vi "GateDelay_Engine_V1.vi"(0 "Port Array":refnum<visa-resource-name>[](array[refnum]), 2 "DelayGate Action":T1=enum."Exit", 5 "Device Index":i32, 9 "Delay Value (steps)":string) -> (8 "Current Delays":i32[][](array[numeric]))   [LabVIEW 2014]
uses:
  GateDelayAction_TypeDef.ctl
  <vilib>/Instr/_visa.llb/VISA Open Access Mode.ctl
  <vilib>/Instr/_visa.llb/VISA Configure Serial Port (Instr).vi
  <vilib>/Instr/_visa.llb/VISA Find Search Mode.ctl
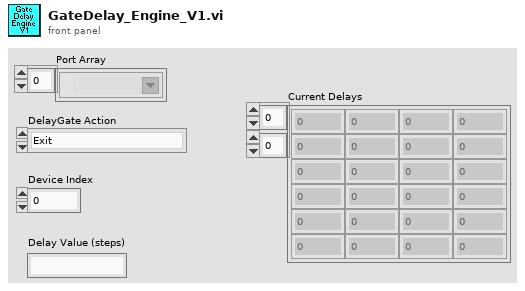
[diagram p1: front panel]
types:
  T1 = typedef "GateDelayAction_TypeDef.ctl" = enum16{"Set Laser Delay", "Set Window Delay", "Set Window Width", "Get Delays", "Exit", "CloseConnections", "Initialize"}
  T2 = typedef "VISA Find Search Mode.ctl" = u32
  T3 = typedef "VISA Open Access Mode.ctl" = u32
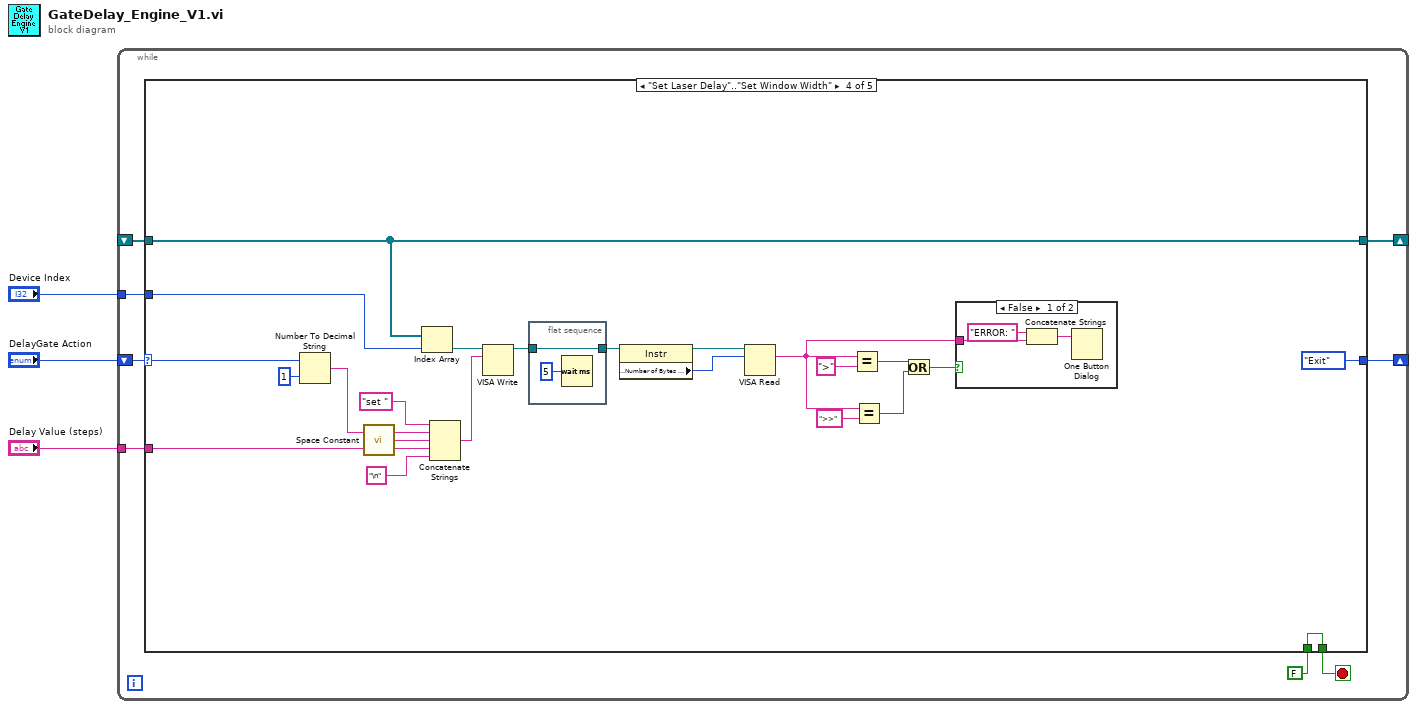
[diagram p0: block diagram]
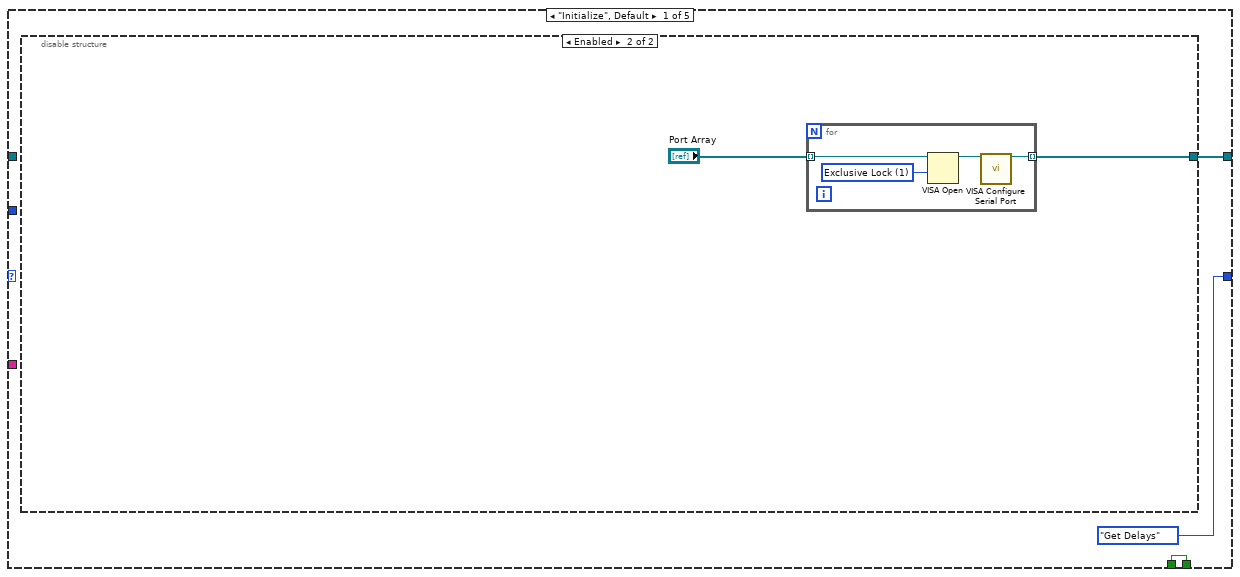
[diagram p2: hidden frame]
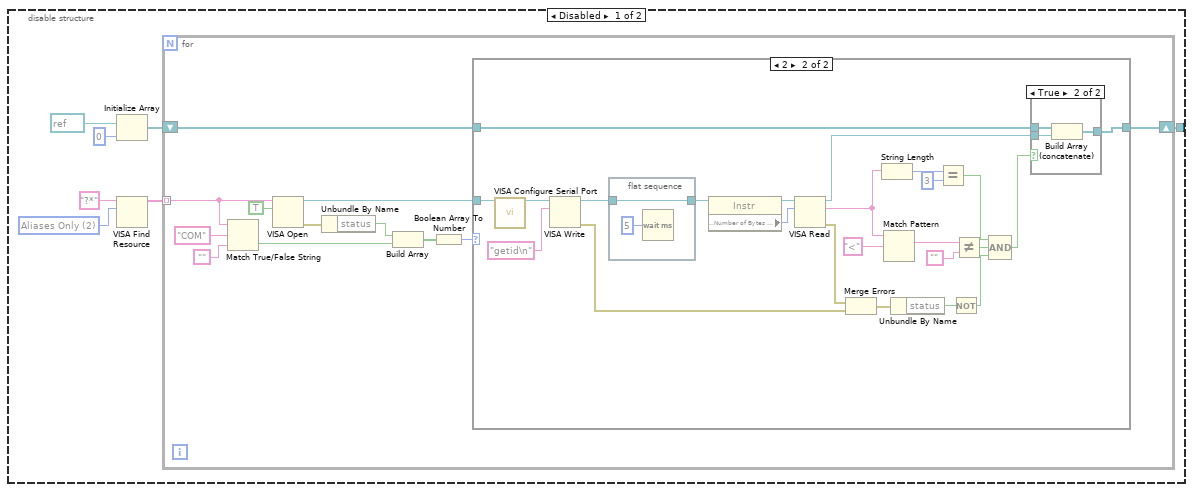
[diagram p3: hidden frame]
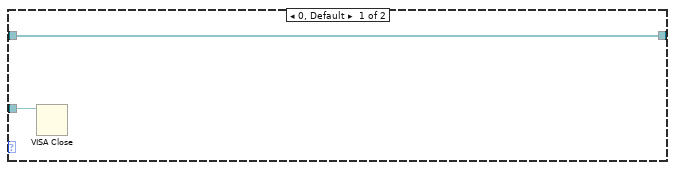
[diagram p4: hidden frame]
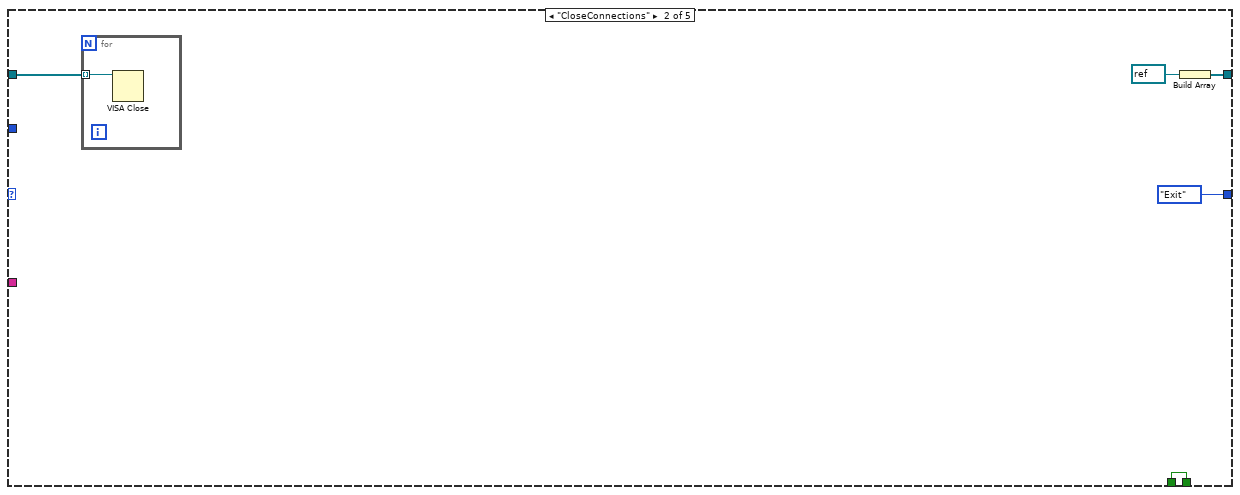
[diagram p6: hidden frame]
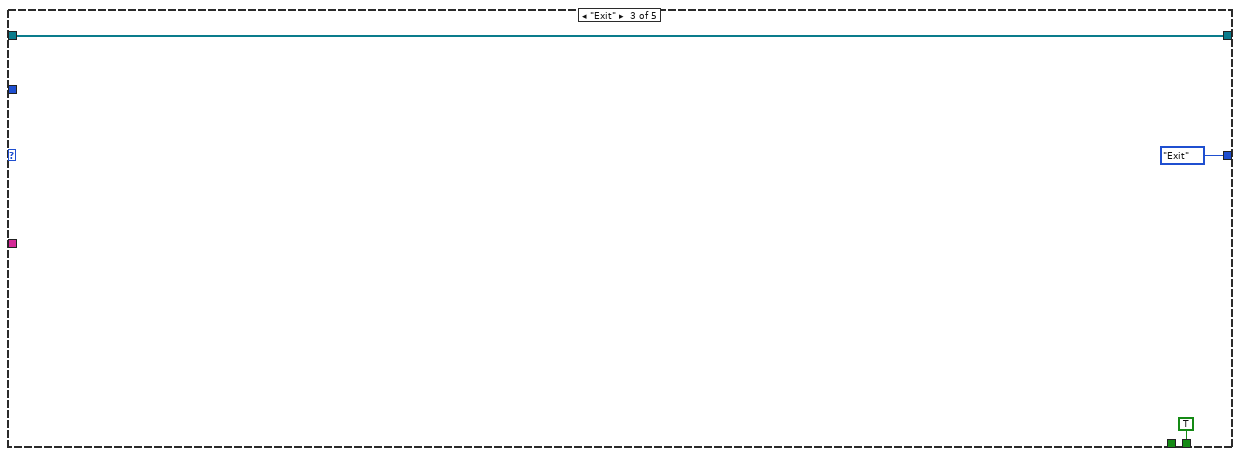
[diagram p7: hidden frame]
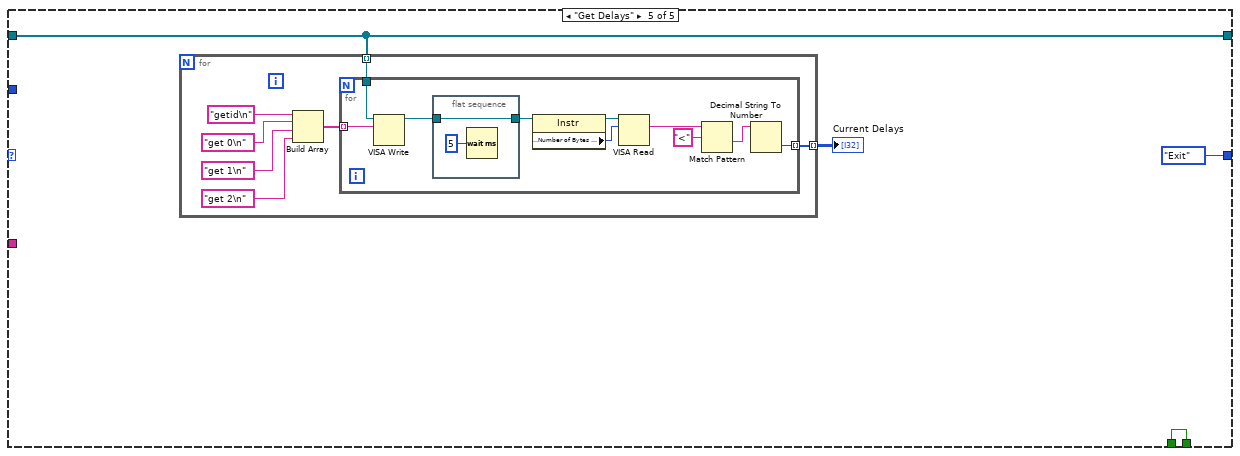
[diagram p9: hidden frame]
diagram:
  n1 = while {
    shift-right: [w8] -> _
    shift-left: "DelayGate Action" -> [w9]
    shift-right: [w11] -> _
    shift-left: _ -> [w10]
    tunnel: "Device Index" -> [w5]
    tunnel: "Delay Value (steps)" -> [w4]
    stop <- w6 stop-if-true
    n2 = case shown="\"Set Laser Delay\"..\"Set Window Width\"" w9 {
      selector: w9 -> [_ _ _ w89 _]
      tunnel: [w14 w73 w78 w103 w110] -> w11
      tunnel: w10 -> [_ w76 w78 w103 w110]
      tunnel: [GateDelayAction_TypeDef."Get Delays" ("Enum") GateDelayAction_TypeDef."Exit" ("Enum") GateDelayAction_TypeDef."Exit" ("Enum") GateDelayAction_TypeDef."Exit" ("Enum") GateDelayAction_TypeDef."Exit" ("Enum")] -> w8
      tunnel: FALSE -> [w12 w72 _ w93 w112]
      tunnel: [w12 w72 TRUE w93 w112] -> w6
      tunnel: w5 -> [_ _ _ w86 _]
      tunnel: w4 -> [_ _ _ w101 _]
      frame "Initialize", Default {
        n3 = disable-structure shown="Enabled" {
          disable-tunnel: [w15 w67] -> w14
          frame Disabled {
            w20 = T2 2 items=["Canonical Names Only"=0, "Aliases Only"=2, "Include Matching Aliases"=3, "Include All Aliases"=4] ("Search Mode")
            n4 = Initialize Array(refnum<visa-resource-name> refnum ("VISA resource name out"), 0 ("dimension size")) -> (w16:refnum<visa-resource-name>[])
            n5 = VISA Find Resource(10:w20, 11:"?*" ("expression (\"?*\")")) -> (3:w19:string[])  [unwired: 1 in, 2 out]
            n6 = for {
              tunnel: w19 -> [w30] mode=indexing
              shift-right: [w23] -> w15
              shift-left: w16 -> [w24]
              n7 = Match True/False String(2:"", 3:"COM" ("true string"), 4:w30) -> (0:w28:bool)  [unwired: 1 out]
              n8 = VISA Open(duplicate session (F)=TRUE, VISA resource name=w30) -> (VISA resource name=w25:refnum<visa-resource-name>, error out=w31:errorcluster)  [unwired: 3 in]
              n9 = Unbundle By Name(w31) -> ("status"=w29:bool)
              n10 = Build Array(w29, w28) -> (w27:bool[])
              n11 = Boolean Array To Number(Boolean array=w27) -> (number=w26:u32)
              n12 = case shown="2" w26 {
                tunnel: w25 -> [w35 w59]
                tunnel: w24 -> [w34 w39]
                tunnel: [w34 w38] -> w23
                frame 0, Default {
                  n13 = VISA Close(VISA resource name=w35) -> ()  [unwired: 1 in, 1 out]
                }
                frame 2 {
                  n14 = call-poly "VISA Configure Serial Port"("VISA resource name"=w59) -> ("VISA resource name out"=w58:refnum<visa-resource-name>)  [unwired: 13 in, 1 out]
                  n15 = VISA Write(VISA resource name=w58, write buffer="getid\n") -> (VISA resource name out=w57:refnum<visa-resource-name>, error out=w45:errorcluster)  [unwired: 1 in, 1 out]
                  n16 = flat-sequence {
                    tunnel: [w65] -> w54
                    tunnel: w57 -> [w65]
                    frame #0 {
                      n17 = Wait (ms)(milliseconds to wait=u32 5) -> ()  [unwired: 1 out]
                    }
                  }
                  n18 = property class="Instr"(reference=w54) -> (reference out=w56:refnum<visa-resource-name>, "Serial Settings:Number of Bytes at Serial Port"=w55:u32)  [unwired: 1 in, 1 out]
                  n19 = VISA Read(VISA resource name=w56, byte count=w55) -> (VISA resource name out=w37:refnum<visa-resource-name>, read buffer=w47:string, error out=w46:errorcluster)  [unwired: 1 in, 1 out]
                  n20 = Merge Errors(w46, w45) -> (w44:errorcluster)
                  n21 = String Length(string=w47) -> (length=w51:i32)
                  n22 = Match Pattern(string=w47, regular expression="<" ("string")) -> (match substring=w50:string)  [unwired: 1 in, 3 out]
                  n23 = Unbundle By Name(w44) -> ("status"=w43:bool)
                  n24 = Equal?(x=w51, y=3) -> (x = y?=w41:bool)
                  n25 = Not(x=w43) -> (.not. x?=w40:bool)
                  n26 = Not Equal?(x=w50, y="") -> (x != y?=w42:bool)
                  n27 = Compound Arithmetic op=AND(w41, w42, w40) -> (w36:bool)
                  n28 = case shown="True" w36 {
                    tunnel: w39 -> [w60 w63]
                    tunnel: [w60 w62] -> w38
                    tunnel: w37 -> [_ w61]
                    frame False {
                    }
                    frame True {
                      n29 = Build Array (concatenate)(w63, w61) -> (w62:refnum<visa-resource-name>[])
                    }
                  }
                }
              }
            }
          }
          frame Enabled {
            n30 = for {
              tunnel: "Port Array" -> [w69] mode=indexing
              tunnel: [w71] -> w67 mode=indexing
              w70 = T3 1 items=["VISA Defaults"=0, "Exclusive Lock"=1, "Load Configured Settings"=4] ("Access Mode")
              n31 = VISA Open(access mode=w70, VISA resource name=w69) -> (VISA resource name=w68:refnum<visa-resource-name>)  [unwired: 3 in, 1 out]
              n32 = call-poly "VISA Configure Serial Port"("VISA resource name"=w68) -> ("VISA resource name out"=w71:refnum<visa-resource-name>)  [unwired: 13 in, 1 out]
            }
          }
        }
      }
      frame "CloseConnections" {
        n33 = for {
          tunnel: w76 -> [w77] mode=indexing
          n34 = VISA Close(VISA resource name=w77) -> ()  [unwired: 1 in, 1 out]
        }
        n35 = Build Array(refnum<visa-resource-name> refnum ("VISA resource name out")) -> (w73:refnum<visa-resource-name>[])
      }
      frame "Exit" {
      }
      frame "Set Laser Delay".."Set Window Width" {
        n36 = Number To Decimal String(number=w89, width (-)=i16 1) -> (decimal integer string=w87:string)
        n37 = call <vilib>:"Space Constant.vi"() -> ("String"=w90:string)
        n38 = Index Array(array=w103, index=w86) -> (element=w102:refnum<visa-resource-name>)
        n39 = Concatenate Strings("set ", w87, w90, w101, "\n") -> (w99:string)
        n40 = VISA Write(VISA resource name=w102, write buffer=w99) -> (VISA resource name out=w96:refnum<visa-resource-name>)  [unwired: 1 in, 2 out]
        n41 = flat-sequence {
          tunnel: [w108] -> w95
          tunnel: w96 -> [w108]
          frame #0 {
            n42 = Wait (ms)(milliseconds to wait=u32 5) -> ()  [unwired: 1 out]
          }
        }
        n43 = property class="Instr"(reference=w95) -> (reference out=w97:refnum<visa-resource-name>, "Serial Settings:Number of Bytes at Serial Port"=w98:u32)  [unwired: 1 in, 1 out]
        n44 = VISA Read(VISA resource name=w97, byte count=w98) -> (read buffer=w82:string)  [unwired: 1 in, 3 out]
        n45 = Equal?(x=w82, y=">") -> (x = y?=w84:bool)
        n46 = Equal?(x=w82, y=">>") -> (x = y?=w83:bool)
        n47 = Or(x=w84, y=w83) -> (x .or. y?=w85:bool)
        n48 = case shown="False" w85 {
          tunnel: w82 -> [w106 _]
          frame False {
            n49 = Concatenate Strings("ERROR: " ("string"), w106) -> (w104:string)
            n50 = One Button Dialog(message=w104) -> ()  [unwired: 1 in, 1 out]
          }
          frame True {
          }
        }
      }
      frame "Get Delays" {
        n51 = for {
          tunnel: [w114] -> w109 mode=indexing
          tunnel: w110 -> [w113] mode=indexing
          n52 = Build Array("getid\n", "get 0\n", "get 1\n", "get 2\n") -> (w115:string[])
          n53 = for {
            tunnel: [w124] -> w114 mode=indexing
            tunnel: w115 -> [w126] mode=indexing
            tunnel: w113 -> [w125]
            n54 = VISA Write(VISA resource name=w125, write buffer=w126) -> (VISA resource name out=w129:refnum<visa-resource-name>)  [unwired: 1 in, 2 out]
            n55 = flat-sequence {
              tunnel: [w131] -> w127
              tunnel: w129 -> [w131]
              frame #0 {
                n56 = Wait (ms)(milliseconds to wait=u32 5) -> ()  [unwired: 1 out]
              }
            }
            n57 = property class="Instr"(reference=w127) -> (reference out=w128:refnum<visa-resource-name>, "Serial Settings:Number of Bytes at Serial Port"=w123:u32)  [unwired: 1 in, 1 out]
            n58 = VISA Read(VISA resource name=w128, byte count=w123) -> (read buffer=w122:string)  [unwired: 1 in, 3 out]
            n59 = Match Pattern(string=w122, regular expression="<") -> (after substring=w120:string)  [unwired: 1 in, 3 out]
            n60 = Decimal String To Number(string=w120) -> (number=w124:i32)  [unwired: 2 in, 1 out]
          }
        }
        "Current Delays" <- w109
      }
    }
  }
